vi "logrecordnumberarray.vi"(7 "logsetting":enum16{"error", "info", "debug"}(ring), 8 "error in":errorcluster, 9 "logtype":enum16{"error", "info", "debug"}(ring), 10 "LogPath":path, 11 "Msg":dbl[](array[numeric])) -> (0 "error out":errorcluster)   [LabVIEW 2011]
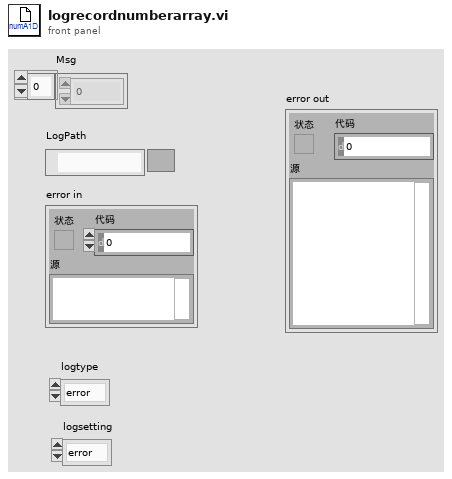
[diagram p1: front panel]
types:
  T1 = enum16{"open", "replace", "create", "open or create", "replace or create", "replace or create with confirmation"}
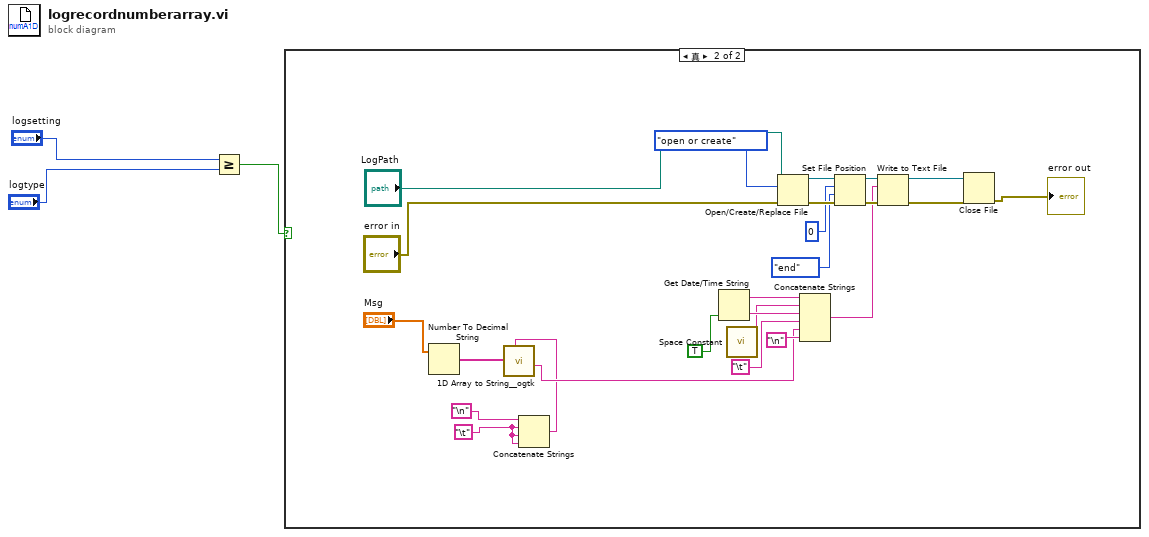
[diagram p0: block diagram]
diagram:
  n1 = Greater Or Equal?(x="logsetting", y="logtype") -> (x >= y?=w1:bool)
  n2 = case shown="真" w1 {
    frame False {
    }
    frame True {
      w5 = "\t"
      n3 = Number To Decimal String(number="Msg") -> (decimal integer string=w8:string[])  [unwired: 1 in]
      n4 = Concatenate Strings("\n", w5, w5, w5) -> (w4:string)
      n5 = call <userlib>:"1D Array to String__ogtk.vi"("delimiter (Tab)"=w4, "Array of Strings"=w8) -> ("delimited string"=w7:string)  [unwired: 9 in]
      n6 = Get Date/Time String(want seconds? (F)=TRUE ("需要秒？(F)")) -> (date string=w14:string, time string=w16:string)  [unwired: 2 in]
      n7 = call <vilib>:"Space Constant.vi"() -> ("String"=w15:string)
      n8 = Open/Create/Replace File(file path (use dialog)="LogPath", error in="error in", operation (0:open)=T1."open or create" ("操作(0:open)")) -> (refnum out=w10:refnum<file>, error out=w21:errorcluster)  [unwired: 3 in, 1 out]
      n9 = Concatenate Strings(w14, w15, w16, "\t", w7, "\n") -> (w19:string)
      n10 = Set File Position(offset (in bytes) (0)=i64 0 ("偏移量（字节）（0）"), refnum=w10, from (0:start)=enum16{"start", "end", "current"}."end" ("自（0:起始）"), error in=w21) -> (refnum out=w12:refnum<file>, error out=w22:errorcluster)
      n11 = Write to Text File(file (use dialog)=w12, text=w19, error in=w22) -> (refnum out=w24:refnum<file>, error out=w25:errorcluster)  [unwired: 1 in, 1 out]
      n12 = Close File(refnum=w24, error in=w25) -> (error out=→"error out":errorcluster)  [unwired: 1 out]
    }
  }
